vi "SSL Detection Robot Referee.vi"(8 "error in":errorcluster, 9 "Array":u8[](array[numeric]) format="%02x") -> (0 "error out":errorcluster, 1 "Length-delimited":u8[](array[numeric]) format="%02x", 3 "output cluster":T1)   [LabVIEW 2023]
uses:
  SSL Referee Team Info.ctl
  Varint Decoder uint32.vi
panel:
  out "string":string
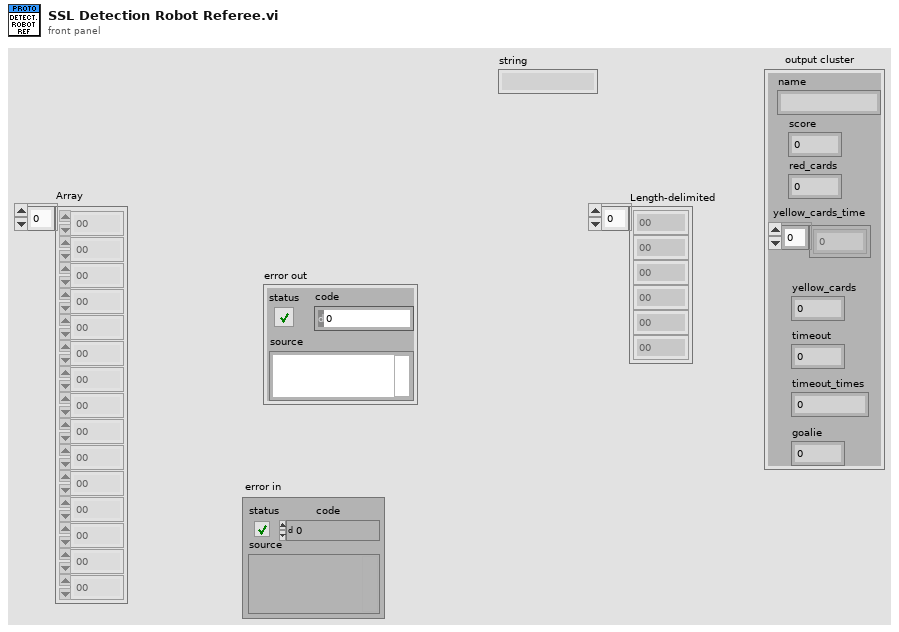
[diagram p1: front panel]
types:
  T1 = typedef "SSL Referee Team Info.ctl" = cluster{"name":string, "score":u32, "red_cards":u32, "yellow_cards_time":u32[], "yellow_cards":u32, "timeout":u32, "timeout_times":u32, "goalie":u32}
  T2 = cluster{"string":string, "Varint":u32, "Varint":u32, u32[], "Varint":u32, "Varint":u32, "Varint":u32, "Varint":u32}
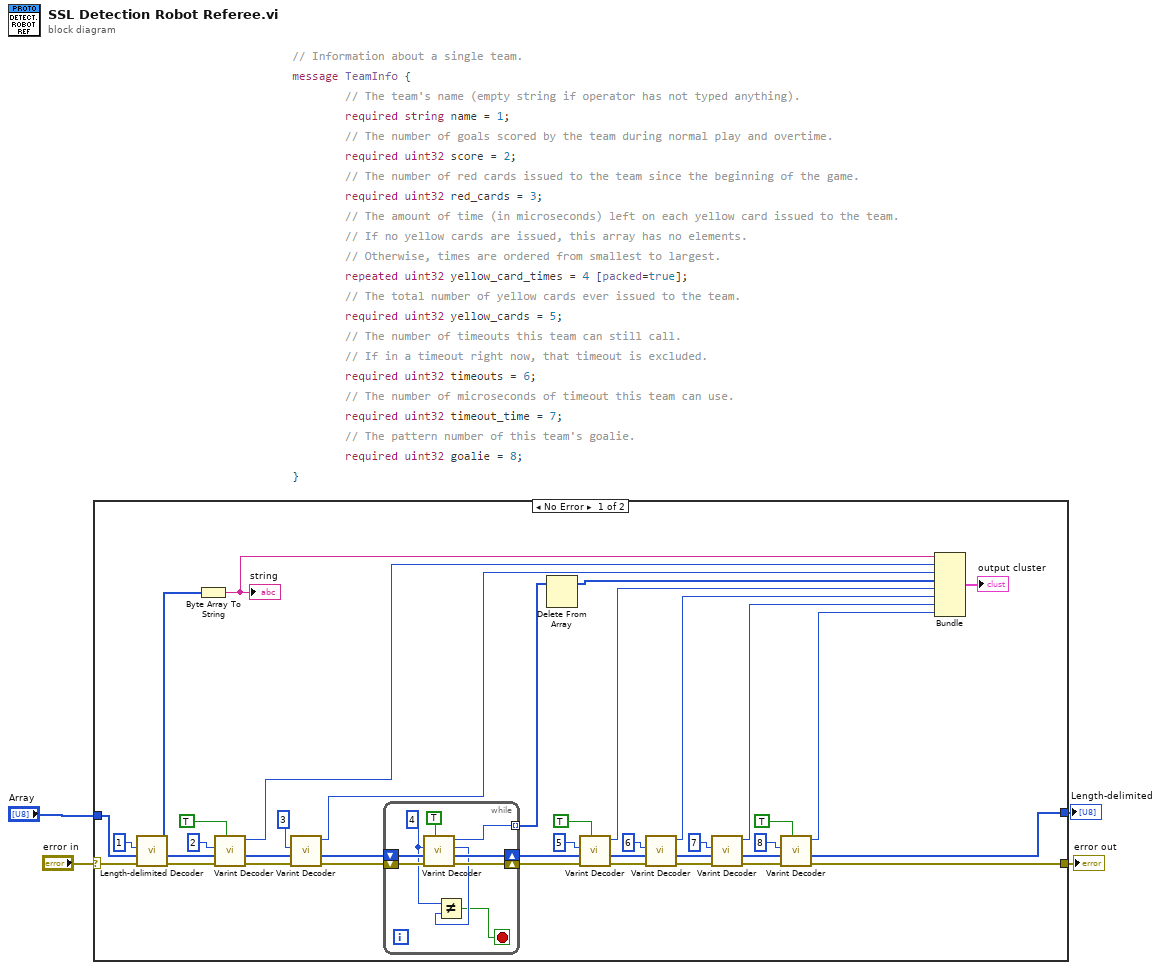
[diagram p0: block diagram]
diagram:
  n1 = case shown="No Error" "error in" {
    selector: "error in" -> [w42 w54]
    tunnel: [w27 w54] -> w3
    tunnel: [w28 w53] -> w2
    tunnel: "Array" -> [w17 w53]
    frame No Error {
      n2 = call "Length-delimited Decoder.vi"("error in (no error)"=w42, "Array"=w17, "Key"=1) -> ("error out"=w41:errorcluster, "array w/ subset deleted"=w16:u8[], "Length-delimited"=w15:u8[])  [unwired: 5 in, 1 out]
      n3 = Byte Array To String(unsigned byte array=w15) -> (string=w14:string)
      "string" <- w14
      n4 = call-poly "Varint Decoder.vi"("Optional"=TRUE, "error in (no error)"=w41, "Array"=w16, "Key"=2) -> ("error out"=w40:errorcluster, "array w/ subset deleted"=w19:u8[], "Varint"=w13:u32)  [unwired: 4 in, 1 out]
      n5 = call-poly "Varint Decoder.vi"("error in (no error)"=w40, "Array"=w19, "Key"=3) -> ("error out"=w39:errorcluster, "array w/ subset deleted"=w20:u8[], "Varint"=w12:u32)  [unwired: 5 in, 1 out]
      n6 = while {
        tunnel: [w49] -> w7 mode=indexing
        shift-right: [w51] -> w35
        shift-left: w39 -> [w52]
        shift-right: [w50] -> w21
        shift-left: w20 -> [w47]
        stop <- w44 stop-if-true
        w46 = 4 ("Key")
        n7 = call-poly "Varint Decoder.vi"("Optional"=TRUE, "error in (no error)"=w52, "Array"=w47, "Key"=w46) -> ("error out"=w51:errorcluster, "array w/ subset deleted"=w50:u8[], "Read Key"=w45:i32, "Varint"=w49:u32)  [unwired: 4 in]
        n8 = Not Equal?(x=w46, y=w45) -> (x != y?=w44:bool)
      }
      n9 = Delete From Array(array=w7) -> (array with subset deleted=w6:u32[])  [unwired: 2 in, 1 out]
      n10 = call-poly "Varint Decoder.vi"("Optional"=TRUE, "error in (no error)"=w35, "Array"=w21, "Key"=5) -> ("error out"=w33:errorcluster, "array w/ subset deleted"=w23:u8[], "Varint"=w11:u32)  [unwired: 4 in, 1 out]
      n11 = call-poly "Varint Decoder.vi"("error in (no error)"=w33, "Array"=w23, "Key"=6) -> ("error out"=w31:errorcluster, "array w/ subset deleted"=w24:u8[], "Varint"=w10:u32)  [unwired: 5 in, 1 out]
      n12 = call-poly "Varint Decoder.vi"("error in (no error)"=w31, "Array"=w24, "Key"=7) -> ("error out"=w29:errorcluster, "array w/ subset deleted"=w25:u8[], "Varint"=w9:u32)  [unwired: 5 in, 1 out]
      n13 = call-poly "Varint Decoder.vi"("Optional"=TRUE, "error in (no error)"=w29, "Array"=w25, "Key"=8) -> ("error out"=w27:errorcluster, "array w/ subset deleted"=w28:u8[], "Varint"=w8:u32)  [unwired: 4 in, 1 out]
      n14 = Bundle("string"=w14, "Varint"=w13, "Varint"=w12, w6, "Varint"=w11, "Varint"=w10, "Varint"=w9, "Varint"=w8) -> (→"output cluster":T2)  [unwired: 1 in]
    }
    frame Error {
    }
  }
  "error out" <- w3
  "Length-delimited" <- w2
